vi "Character Count Limit Reached.vi"(6 "Character Count Limit Reached":bool, 7 "Full String":string, 9 "Response In":string, 10 "Remaining string in":string) -> (1 "Response out":string, 2 "Remaining string out":string)   [LabVIEW 2017, in "SSH.lvlib"]
doc: "If the Character count limit has been reached, output the entire buffer string and set the remaining string to be empty"
uses:
  SSH.lvlib
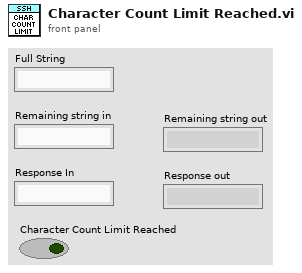
[diagram p1: front panel]
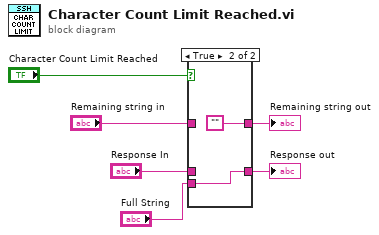
[diagram p0: block diagram]
diagram:
  n1 = case shown="True" "Character Count Limit Reached" {
    tunnel: "Remaining string in" -> [w8 _]
    tunnel: [w8 ""] -> w3
    tunnel: [w7 w10] -> w4
    tunnel: "Response In" -> [w7 _]
    tunnel: "Full String" -> [_ w10]
    frame False {
    }
    frame True {
    }
  }
  "Response out" <- w4
  "Remaining string out" <- w3
